vi "Close.vi"(8 "error in (no error)":errorcluster {"code" format="Error %.0f"}, 11 "VIDoc Parser In":refnum<class "VIDoc Parser.lvclass">) -> (0 "error out":errorcluster {"code" format="Error %.0f"})   [LabVIEW 2023, in "VIDoc Parsing.lvlib" / "VIDoc Parser.lvclass"]
uses:
  VIDoc Parser.lvclass
  VIDoc Parser.lvclass/VIDoc Parser.ctl
  UI Interaction/UI Interaction.lvclass
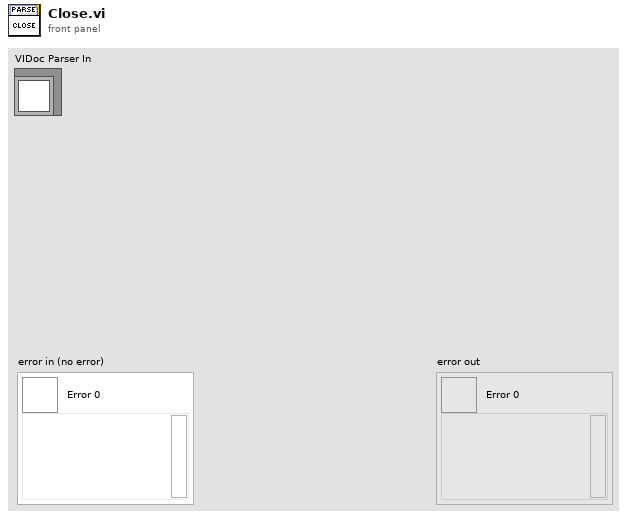
[diagram p1: front panel]
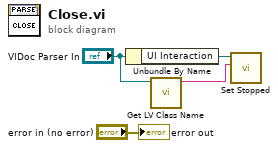
[diagram p0: block diagram]
diagram:
  n1 = Unbundle By Name("VIDoc Parser In") -> ("UI Interaction"=w4:refnum<class "UI Interaction.lvclass">)
  n2 = call <vilib>:"Get LV Class Name.vi"("object"="VIDoc Parser In") -> ("class name"=w1:string)  [unwired: 9 in, 1 out]
  n3 = call-dynamic "Set Stopped.vi"("Process"=w1, "UI Interaction in"=w4) -> ()  [unwired: 8 in, 2 out]
  "error out" <- "error in (no error)"
